vi "get_script_body_test.vi"() -> ()   [LabVIEW 2017, in "labview-standard-library.lvlib" / "automode-scripting.lvlib"]
uses:
  automode-scripting.lvlib
panel:
  out "x = y?":bool
  out "Script Body":string[](array[string])
  out "Full Text":string
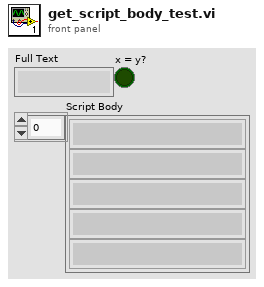
[diagram p1: front panel]
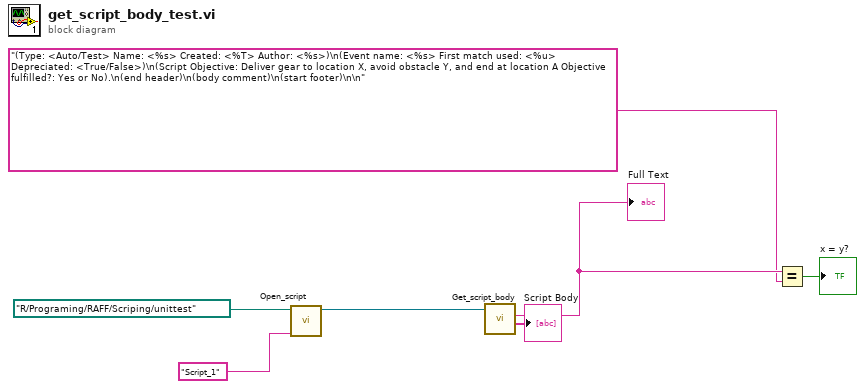
[diagram p0: block diagram]
diagram:
  n1 = call "Open_script.vi"("Script name"="Script_1", "Folder Path"=path "R:/Programing/RAFF/Scriping/unittest") -> ("Byte Stream File out"=w5:refnum<file>)  [unwired: 8 in, 1 out]
  n2 = call "Get_script_body.vi"("Byte Stream File in"=w5) -> ("Script Body"=→"Script Body":string[], "Full Text"=w4:string)  [unwired: 8 in, 1 out]
  "Full Text" <- w4
  n3 = Equal?(x=w4, y="(Type: <Auto/Test> Name: <%s> Created: <%T> Author: <%s>)\n(Event name: <%s> First match used: <%u> Depreciated: <True/False>)\n(Script Objective: Deliver gear to location X, avoid obstacle Y, and end at location A Objective fulfilled?: Yes or No).\n(end header)\n(body comment)\n(start footer)\n\n") -> (x = y?=→"x = y?":bool)
